vi "GetUserGroupLevel.vi"(8 "error in (no error)":errorcluster, 11 "user":string) -> (0 "error out":errorcluster, 3 "user level":i32)   [LabVIEW 2019]
uses:
  LVWinFun.dll
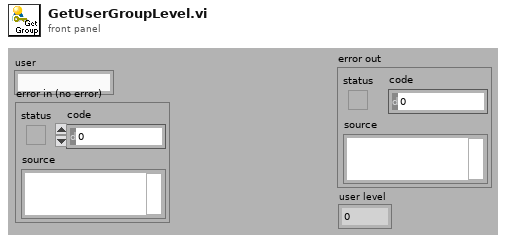
[diagram p1: front panel]
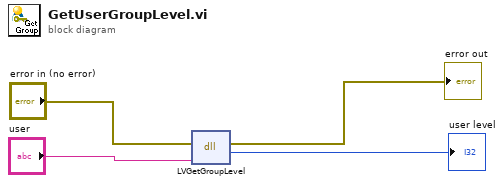
[diagram p0: block diagram]
diagram:
  n1 = dll-call lib="F:/src/HUTCDLSVN/Machine/CDL0100/HMI/Support VIs/LVWinFun.dll" fn="LVGetGroupLevel"(error in="error in (no error)", "user"="user") -> (error out=→"error out":errorcluster, "user level"=→"user level":i32)  [unwired: 3 in, 1 out]
